vi "Read Mode.vi"(8 "error in (no error)":errorcluster, 11 "RFSoC Driver in":refnum<class "RFSoC Driver.lvclass">) -> (0 "error out":errorcluster, 2 "Mode":enum16{"Pulse", "Sine"}(ring), 3 "RFSoC Driver out":refnum<class "RFSoC Driver.lvclass">)   [LabVIEW 2019, in "RFSoC Driver.lvclass"]
uses:
  RFSoC Driver.lvclass
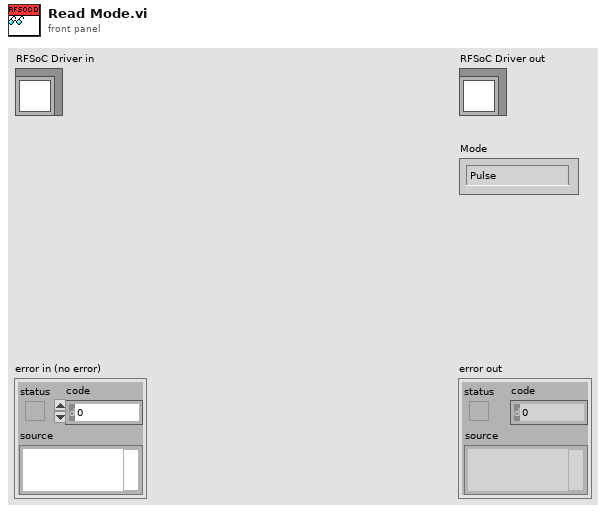
[diagram p1: front panel]
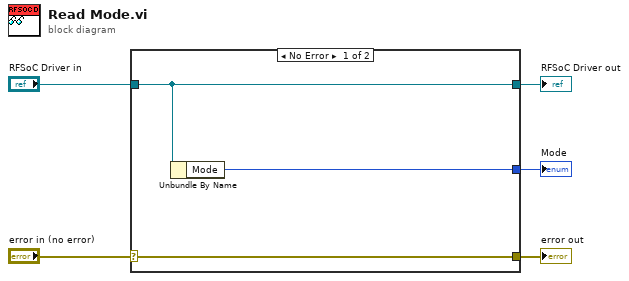
[diagram p0: block diagram]
diagram:
  n1 = case shown="No Error" "error in (no error)" {
    selector: "error in (no error)" -> [w8 w9]
    tunnel: [w8 w9] -> w4
    tunnel: [w7 w10] -> w2
    tunnel: "RFSoC Driver in" -> [w7 w10]
    tunnel: [w6 _] -> w1
    frame No Error {
      n2 = Unbundle By Name(w7) -> ("Mode"=w6:enum16{"Pulse", "Sine"})
    }
    frame Error {
    }
  }
  "error out" <- w4
  "RFSoC Driver out" <- w2
  "Mode" <- w1
